vi "fpgastart.vi"() -> (0 "FPGA VI Reference Out":refnum<k20>)   [LabVIEW 2010]
uses:
  <vilib>/rvi/interface/nirviOpenFPGA/nirviOpenFPGA.xnode
  C:/Users/HAGAR-IV/Desktop/Zeugs/Johnny/pertrasgc fpga/fpga-programm-2.vi
  <vilib>/userDefined/High Color/nirio_resource_hc.ctl
  <vilib>/rvi/interface/nirviReadWriteControl/nirviReadWriteControl.xnode
  <vilib>/rvi/errors/niLvFpgaWhatHappensToTopLevelVI.ctl
  <vilib>/rvi/interface/common/niFpgaNodeNameForErrorReporting.ctl
  <vilib>/rvi/errors/niLvFpgaAdjustHostInterfaceError.vi
  <vilib>/rvi/interface/nirviMethod/nirviMethod.xnode
  <vilib>/LabVIEW Targets/FPGA/cRIO/shared/nicrio_ModuleControls/nicrio_cRIO-9871_BaudRateEnum.ctl
  <vilib>/LabVIEW Targets/FPGA/cRIO/shared/nicrio_ModuleControls/nicrio_cRIO-9871_DataBitsEnum.ctl
  <vilib>/LabVIEW Targets/FPGA/cRIO/shared/nicrio_ModuleControls/nicrio_cRIO-9871_ParityEnum.ctl
  <vilib>/LabVIEW Targets/FPGA/cRIO/shared/nicrio_ModuleControls/nicrio_cRIO-9871_StopBitsEnum.ctl
  <vilib>/LabVIEW Targets/FPGA/cRIO/shared/nicrio_ModuleControls/nicrio_cRIO-9871_FlowControlEnum.ctl
  <vilib>/RVI Host/nirviSupport.llb/nirviErrorClusterFromErrorCode.vi
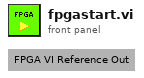
[diagram p1: front panel]
types:
  T1 = cluster{"PIDMach1":cluster{"proportional gain (Kc)":fxp<+/-,16,8>, "integral gain (Kc*Ts/Ti)":fxp<+/-,16,8>, "derivative gain (Kc*Td/Ts)":fxp<+/-,16,8>}, "Umax[V]Mach1":fxp<+/-,16,4>, "Heizen?Mach1":bool, "USetp[V]Mach1":fxp<+/-,16,4>, "PIDMach2":cluster{"proportional gain (Kc)":fxp<+/-,16,8>, "integral gain (Kc*Ts/Ti)":fxp<+/-,16,8>, "derivative gain (Kc*Td/Ts)":fxp<+/-,16,8>}, "Umax[V]Mach2":fxp<+/-,16,4>, "Heizen?Mach2":bool, "USetp[V]Mach2":fxp<+/-,16,4>}
  T2 = cluster{"PIDTrap2":cluster{"proportional gain (Kc)":fxp<+/-,16,8>, "integral gain (Kc*Ts/Ti)":fxp<+/-,16,8>, "derivative gain (Kc*Td/Ts)":fxp<+/-,16,8>}, "UTempMaxTrap2":fxp<+/-,16,4>, "UWidrMaxTrap2":fxp<+/-,16,4>, "Heizen?Trap2":bool, "UTempSPTrap2":fxp<+/-,16,4>}
  T3 = cluster{"PIDTrap1":cluster{"proportional gain (Kc)":fxp<+/-,16,8>, "integral gain (Kc*Ts/Ti)":fxp<+/-,16,8>, "derivative gain (Kc*Td/Ts)":fxp<+/-,16,8>}, "UTempMaxTrap1":fxp<+/-,16,4>, "UWidrMaxTrap1":fxp<+/-,16,4>, "Heizen?Trap1":bool, "UTempSPTrap1":fxp<+/-,16,4>}
  T4 = cluster{"Per[us]Trap1":u32, "warten[us]Trap1":u32, "Per[us]Trap2":u32, "warten[us]Trap2":u32, "Per[us]Mach":u16, "vor der Messung [us]Mach":u16, "wie viele Messwerte?Mach":u16, "Abstand zwischen Messungen [us]Mach":u16}
  T5 = typedef "nicrio_cRIO-9871_BaudRateEnum.ctl" = enum16{"75 bps", "110 bps", "134 bps", "150 bps", "300 bps", "600 bps", "1200 bps", "1800 bps", "2400 bps", "4800 bps", "7200 bps", "9600 bps", "14.4 kbps", "19.2 kbps", "28.8 kbps", "38.4 kbps", "57.6 kbps", "115.2 kbps", "230.4 kbps", "460.8 kbps", "921.6 kbps"}
  T6 = typedef "nicrio_cRIO-9871_DataBitsEnum.ctl" = enum8{"5", "6", "7", "8"}
  T7 = typedef "nicrio_cRIO-9871_ParityEnum.ctl" = enum8{"None", "Odd", "Even", "Mark", "Space"}
  T8 = typedef "nicrio_cRIO-9871_StopBitsEnum.ctl" = enum8{"1", "1.5", "2"}
  T9 = typedef "nicrio_cRIO-9871_FlowControlEnum.ctl" = enum8{"None", "Software (XON / XOFF)", "Hardware (RTS / CTS)"}
  T10 = cluster{"Mod7/Port1":cluster{"Baud Rate":T5, "Data Bits":T6, "Parity":T7, "Stop Bits":T8, "Flow Control":T9}, "Mod7/Port2":cluster{"Baud Rate":T5, "Data Bits":T6, "Parity":T7, "Stop Bits":T8, "Flow Control":T9}, "Mod7/Port3":cluster{"Baud Rate":T5, "Data Bits":T6, "Parity":T7, "Stop Bits":T8, "Flow Control":T9}, "Mod7/Port4":cluster{"Baud Rate":T5, "Data Bits":T6, "Parity":T7, "Stop Bits":T8, "Flow Control":T9}, "Mod8/Port1":cluster{"Baud Rate":T5, "Data Bits":T6, "Parity":T7, "Stop Bits":T8, "Flow Control":T9}, "Mod8/Port2":cluster{"Baud Rate":T5, "Data Bits":T6, "Parity":T7, "Stop Bits":T8, "Flow Control":T9}, "Mod8/Port3":cluster{"Baud Rate":T5, "Data Bits":T6, "Parity":T7, "Stop Bits":T8, "Flow Control":T9}, "Mod8/Port4":cluster{"Baud Rate":T5, "Data Bits":T6, "Parity":T7, "Stop Bits":T8, "Flow Control":T9}}
  T11 = cluster{"ServoTrap1kalt":bool, "Servo1WarmHigh(us)":u32, "Servo1KaltHigh(us)":u32, "ServoTrap2kalt":bool, "Servo2WarmHigh(us)":u32, "Servo2KaltHigh(us)":u32}
  T12 = cluster{"Bronkhorst1":bool, "Bronkhorst1 ":u16, "MainCol1":bool, "MainCol1":u16, "MainCol2":bool, "MainCol2":u16, "Bronkhorst2":bool, "Bronkhorst2":u16, "Oven":bool, "Oven":u16, "T-Line":bool, "T-Line":u16}
  T13 = cluster{"Mod6/DIO0":bool, "Mod6/DIO3":bool, "Mod6/DIO4":bool, "Mod6/DIO5":bool, "Mod6/DIO6":bool, "Mod6/DIO7":bool, "Mod6/DIO8":bool, "Mod6/DIO9":bool, "Mod6/DIO10":bool, "Mod6/DIO11":bool, "Mod6/DIO12":bool, "Mod6/DIO13":bool, "Mod6/DIO14":bool, "Mod6/DIO15":bool, "Mod6/DIO16":bool, "Mod6/DIO17":bool, "Mod6/DIO18":bool, "Mod6/DIO19":bool, "Mod6/DIO20":bool, "Mod6/DIO21":bool, "Mod6/DIO22":bool, "Mod6/DIO23":bool, "Mod6/DIO24":bool, "Mod6/DIO25":bool, "Mod6/DIO26":bool, "Mod6/DIO27":bool, "Mod6/DIO28":bool, "Mod6/DIO29":bool, "Mod6/DIO30":bool, "Mod6/DIO31":bool}
  T14 = cluster{"Mod5/DIO5":bool, "Mod5/DIO6":bool, "Mod5/DIO7":bool, "Mod5/DIO10":bool, "Mod5/DIO11":bool, "Mod5/DIO14":bool, "Mod5/DIO15":bool, "Mod5/DIO16":bool, "Mod5/DIO17":bool, "Mod5/DIO18":bool, "Mod5/DIO20":bool, "Mod5/DIO23":bool, "Mod5/DIO25":bool, "Mod5/DIO26":bool, "Mod5/DIO27":bool, "Mod5/DIO28":bool, "Mod5/DIO29":bool, "Mod5/DIO30":bool}
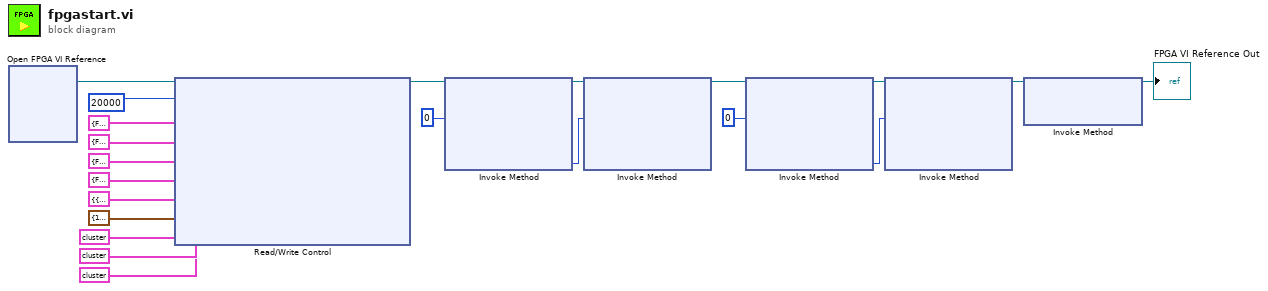
[diagram p0: block diagram]
diagram:
  n1 = xnode "Open FPGA VI Reference"() -> ("FPGA VI Reference Out"=w21:refnum<k20>)  [unwired: 2 in, 1 out]
  n2 = xnode "Read/Write Control"("FPGA VI Reference In"=w21, "ServosPeriode(us)"=u32 20000, "Mod5/DIOs"=T14 {"Mod5/DIO5"=FALSE, "Mod5/DIO6"=FALSE, "Mod5/DIO7"=FALSE, "Mod5/DIO10"=FALSE, "Mod5/DIO11"=FALSE, "Mod5/DIO14"=FALSE, "Mod5/DIO15"=FALSE, "Mod5/DIO16"=FALSE, "Mod5/DIO17"=FALSE, "Mod5/DIO18"=FALSE, "Mod5/DIO20"=FALSE, "Mod5/DIO23"=FALSE, "Mod5/DIO25"=FALSE, "Mod5/DIO26"=FALSE, "Mod5/DIO27"=FALSE, "Mod5/DIO28"=FALSE, "Mod5/DIO29"=FALSE, "Mod5/DIO30"=FALSE}, "Mod6/DIOs"=T13 {"Mod6/DIO0"=FALSE, "Mod6/DIO3"=FALSE, "Mod6/DIO4"=FALSE, "Mod6/DIO5"=FALSE, "Mod6/DIO6"=FALSE, "Mod6/DIO7"=FALSE, "Mod6/DIO8"=FALSE, "Mod6/DIO9"=FALSE, "Mod6/DIO10"=FALSE, "Mod6/DIO11"=FALSE, "Mod6/DIO12"=FALSE, "Mod6/DIO13"=FALSE, "Mod6/DIO14"=FALSE, "Mod6/DIO15"=FALSE, "Mod6/DIO16"=FALSE, "Mod6/DIO17"=FALSE, "Mod6/DIO18"=FALSE, "Mod6/DIO19"=FALSE, "Mod6/DIO20"=FALSE, "Mod6/DIO21"=FALSE, "Mod6/DIO22"=FALSE, "Mod6/DIO23"=FALSE, "Mod6/DIO24"=FALSE, "Mod6/DIO25"=FALSE, "Mod6/DIO26"=FALSE, "Mod6/DIO27"=FALSE, "Mod6/DIO28"=FALSE, "Mod6/DIO29"=FALSE, "Mod6/DIO30"=FALSE, "Mod6/DIO31"=FALSE}, "LH Heizen? Pulse (us)"=T12 {"Bronkhorst1"=FALSE, "Bronkhorst1 "=0, "MainCol1"=FALSE, "MainCol1"=0, "MainCol2"=FALSE, "MainCol2"=0, "Bronkhorst2"=FALSE, "Bronkhorst2"=0, "Oven"=FALSE, "Oven"=0, "T-Line"=FALSE, "T-Line"=0}, "Servos kalt? WarmHigh (us) KaltHigh (us)"=T11 {"ServoTrap1kalt"=FALSE, "Servo1WarmHigh(us)"=0, "Servo1KaltHigh(us)"=0, "ServoTrap2kalt"=FALSE, "Servo2WarmHigh(us)"=0, "Servo2KaltHigh(us)"=0}, "KonfigSeriell"=T10 {"Mod7/Port1"={"Baud Rate"=enum."38.4 kbps", "Data Bits"=enum."8", "Parity"=enum."None", "Stop Bits"=enum."1", "Flow Control"=enum."None"}, "Mod7/Port2"={"Baud Rate"=enum."38.4 kbps", "Data Bits"=enum."8", "Parity"=enum."None", "Stop Bits"=enum."1", "Flow Control"=enum."None"}, "Mod7/Port3"={"Baud Rate"=enum."38.4 kbps", "Data Bits"=enum."8", "Parity"=enum."None", "Stop Bits"=enum."1", "Flow Control"=enum."None"}, "Mod7/Port4"={"Baud Rate"=enum."38.4 kbps", "Data Bits"=enum."8", "Parity"=enum."None", "Stop Bits"=enum."1", "Flow Control"=enum."None"}, "Mod8/Port1"={"Baud Rate"=enum."38.4 kbps", "Data Bits"=enum."8", "Parity"=enum."None", "Stop Bits"=enum."1", "Flow Control"=enum."None"}, "Mod8/Port2"={"Baud Rate"=enum."38.4 kbps", "Data Bits"=enum."8", "Parity"=enum."None", "Stop Bits"=enum."1", "Flow Control"=enum."None"}, "Mod8/Port3"={"Baud Rate"=enum."38.4 kbps", "Data Bits"=enum."8", "Parity"=enum."None", "Stop Bits"=enum."1", "Flow Control"=enum."None"}, "Mod8/Port4"={"Baud Rate"=enum."38.4 kbps", "Data Bits"=enum."8", "Parity"=enum."None", "Stop Bits"=enum."1", "Flow Control"=enum."None"}}, "SHFest"=T4 {"Per[us]Trap1"=10000, "warten[us]Trap1"=2000, "Per[us]Trap2"=10000, "warten[us]Trap2"=2000, "Per[us]Mach"=20000, "vor der Messung [us]Mach"=600, "wie viele Messwerte?Mach"=14, "Abstand zwischen Messungen [us]Mach"=150}, "Trap1"=T3 {"PIDTrap1"={"proportional gain (Kc)"=0.0, "integral gain (Kc*Ts/Ti)"=0.0, "derivative gain (Kc*Td/Ts)"=0.0}, "UTempMaxTrap1"=0.0, "UWidrMaxTrap1"=0.0, "Heizen?Trap1"=FALSE, "UTempSPTrap1"=0.0}, "Trap2"=T2 {"PIDTrap2"={"proportional gain (Kc)"=0.0, "integral gain (Kc*Ts/Ti)"=0.0, "derivative gain (Kc*Td/Ts)"=0.0}, "UTempMaxTrap2"=0.0, "UWidrMaxTrap2"=0.0, "Heizen?Trap2"=FALSE, "UTempSPTrap2"=0.0}, "Machs"=T1 {"PIDMach1"={"proportional gain (Kc)"=0.0, "integral gain (Kc*Ts/Ti)"=0.0, "derivative gain (Kc*Td/Ts)"=0.0}, "Umax[V]Mach1"=0.0, "Heizen?Mach1"=FALSE, "USetp[V]Mach1"=0.0, "PIDMach2"={"proportional gain (Kc)"=0.0, "integral gain (Kc*Ts/Ti)"=0.0, "derivative gain (Kc*Td/Ts)"=0.0}, "Umax[V]Mach2"=0.0, "Heizen?Mach2"=FALSE, "USetp[V]Mach2"=0.0}) -> ("FPGA VI Reference Out"=w20:refnum<k20>)  [unwired: 1 in, 1 out]
  n3 = xnode "Invoke Method"("FPGA VI Reference In"=w20, "Number of Elements"=u32 0) -> ("FPGA VI Reference Out"=w19:refnum<k20>, "Elements Remaining"=w13:u32)  [unwired: 2 in, 2 out]
  n4 = xnode "Invoke Method"("FPGA VI Reference In"=w19, "Number of Elements"=w13) -> ("FPGA VI Reference Out"=w18:refnum<k20>)  [unwired: 2 in, 3 out]
  n5 = xnode "Invoke Method"("FPGA VI Reference In"=w18, "Number of Elements"=u32 0) -> ("FPGA VI Reference Out"=w17:refnum<k20>, "Elements Remaining"=w11:u32)  [unwired: 2 in, 2 out]
  n6 = xnode "Invoke Method"("FPGA VI Reference In"=w17, "Number of Elements"=w11) -> ("FPGA VI Reference Out"=w16:refnum<k20>)  [unwired: 2 in, 3 out]
  n7 = xnode "Invoke Method"("FPGA VI Reference In"=w16) -> ("FPGA VI Reference Out"=→"FPGA VI Reference Out":refnum<k20>)  [unwired: 2 in, 1 out]
